vi "XDimension conversion.vi"(11 "Input XDimension":string) -> (2 "Enum Control Value":i32, 3 "Output XDimension":string)   [LabVIEW 2020, in "GetSetShared.lvlib"]
uses:
  <vilib>/express/express signal manip/GetorSetDDTAttributes/Shared VIs/GetSetShared.lvlib
  <vilib>/express/express signal manip/GetorSetDDTAttributes/Shared VIs/XDimension.ctl
panel:
  in  "XDimension Enum":T1=enum."Time [sec]" caption="Value"
  in  "XDimension 1":string[](array[string])=["No X Unit [-]", "Time [sec]", "Frequency [Hz]"]
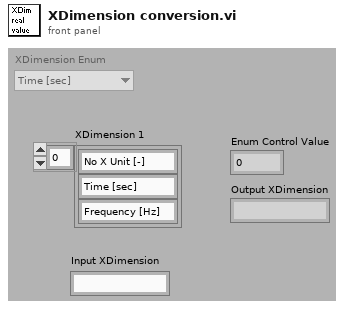
[diagram p1: front panel]
types:
  T1 = typedef "GetSetShared.lvlib/XDimension.ctl" = enum16{"No Unit [-]", "Time [sec]", "Frequency [Hz]"}
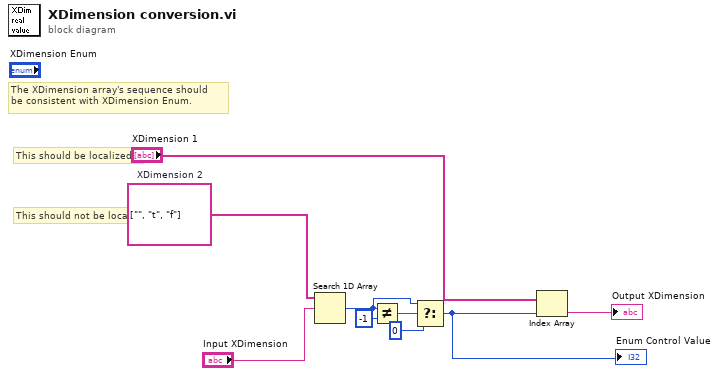
[diagram p0: block diagram]
diagram:
  w7 = string[] ["", "t", "f"]  # XDimension 2
  # "This should not be localized"
  # "This should be localized"
  # "The XDimension array's sequence should\nbe consistent with XDimension Enum."
  n1 = Search 1D Array(1D array=w7, element="Input XDimension") -> (index of element=w3:i32)  [unwired: 1 out]
  n2 = Not Equal?(x=w3, y=-1) -> (x != y?=w4:bool)
  n3 = Select(t=w3, s=w4, f=0) -> (s? t:f=w1:i32)
  "Enum Control Value" <- w1
  n4 = Index Array(array="XDimension 1", index=w1) -> (element=→"Output XDimension":string)
